vi "Lab0.vi"() -> ()   [LabVIEW 2010]
panel:
  in  "ON/OFF":bool
  in  "stop":bool
  out "Text":string
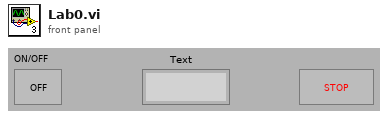
[diagram p1: front panel]
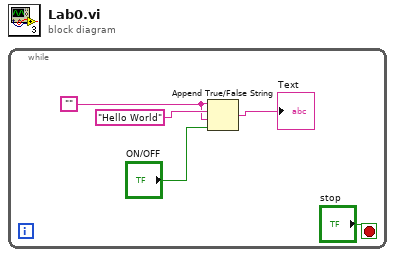
[diagram p0: block diagram]
diagram:
  n1 = while {
    stop <- "stop" stop-if-true
    w2 = ""
    n2 = Append True/False String(1:"ON/OFF", 2:w2, 3:"Hello World" ("String"), 4:w2) -> (0:→"Text":string)
  }
